vi "st_Neg Binomial Inverse CDF (kx).vi"(9 "p":dbl=0.4, 10 "x":dbl=10.0, 11 "cdf(y)":dbl=0.5) -> (0 "error":i32, 3 "y":dbl=5.775864720810446)   [LabVIEW 2018, in "NI_Gmath.lvlib"]
uses:
  NI_Gmath.lvlib
  st_error_code.ctl
panel:
  # "Negative Binomial Inverse CDF"
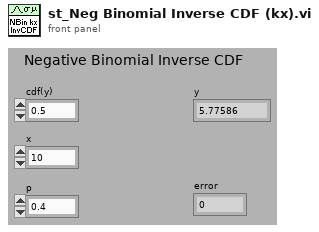
[diagram p1: front panel]
types:
  T1 = typedef "NI_Gmath.lvlib/st_error_code.ctl" = i32
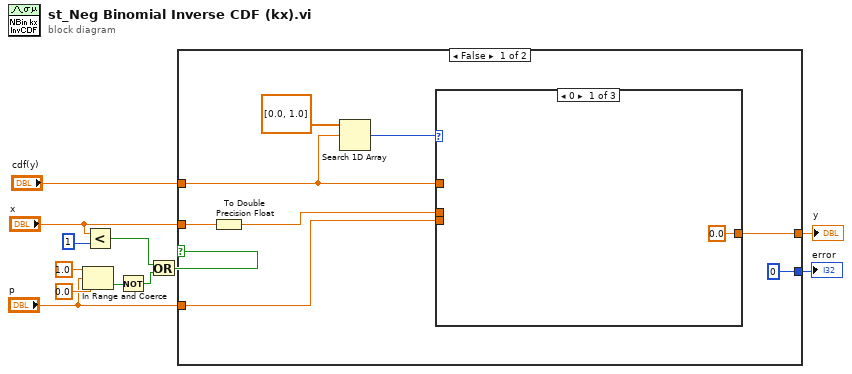
[diagram p0: block diagram]
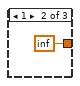
[diagram p2: hidden frame]
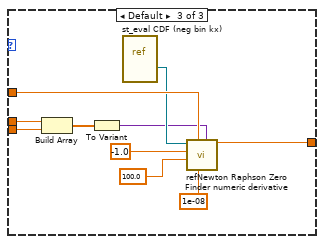
[diagram p3: hidden frame]
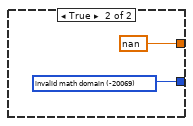
[diagram p4: hidden frame]
diagram:
  n1 = In Range and Coerce(upper limit=1.0, x="p", lower limit=0.0) -> (In Range?=w7:bool)  [unwired: 1 out]
  n2 = Less?(x="x", y=1) -> (x < y?=w5:bool)
  n3 = Not(x=w7) -> (.not. x?=w6:bool)
  n4 = Or(x=w5, y=w6) -> (x .or. y?=w1:bool)
  n5 = case shown="False" w1 {
    tunnel: "p" -> [w18 _]
    tunnel: [0 ("invalid math domain") w33] -> w12
    tunnel: [w17 nan] -> w11
    tunnel: "cdf(y)" -> [w15 _]
    tunnel: "x" -> [w19 _]
    frame False {
      n6 = To Double Precision Float(number=w19) -> (double precision float=w13:dbl)
      n7 = Search 1D Array(1D array=dbl[] [0.0, 1.0], element=w15) -> (index of element=w14:i32)  [unwired: 1 in]
      n8 = case shown="0" w14 {
        tunnel: w13 -> [_ _ w31]
        tunnel: w18 -> [_ _ w30]
        tunnel: [0.0 ("zero") inf ("zero") w29] -> w17
        tunnel: w15 -> [_ _ w25]
        frame 0 {
        }
        frame 1 {
        }
        frame Default {
          n9 = Build Array(w31, w30) -> (w32:dbl[])
          n10 = To Variant(anything=w32) -> (Variant=w23:variant)
          n11 = vi-ref "st_eval CDF (neg bin kx).vi"() -> ("vi reference"=w24:refnum<vi>)
          n12 = call "refNewton Raphson Zero Finder numeric derivative.vi"("function parameters"=w23, "accuracy"=1e-08, "level"=w25, "end"=100.0, "start"=-1.0, "function refnum"=w24) -> ("zero"=w29:dbl)  [unwired: 2 in, 3 out]
        }
      }
    }
    frame True {
      w33 = T1 -20069 items=["invalid math domain"=-20069, "Fourier interpolation size m >= n"=-20070, "empty array"=-20003] ("stat interp error code")
    }
  }
  "y" <- w11
  "error" <- w12
